vi "Begin Map by Reference.vi"(8 "Error In":errorcluster, 11 "Reader In":refnum<data-value>) -> (0 "Error Out":errorcluster, 2 "Count":u32, 3 "Reader Out":refnum<data-value>)   [LabVIEW 2017, in "LabPack.lvlib" / "Reader.lvclass"]
uses:
  Reader.lvclass
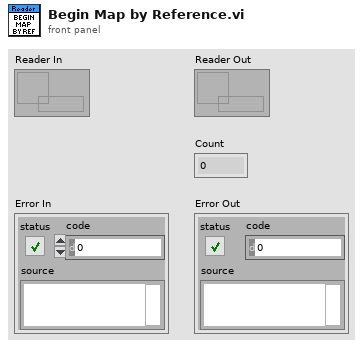
[diagram p1: front panel]
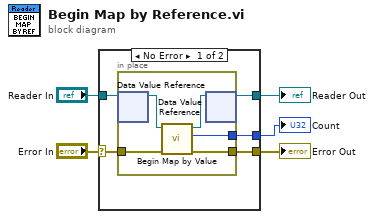
[diagram p0: block diagram]
diagram:
  n1 = case shown="No Error" "Error In" {
    selector: "Error In" -> [w8 w16]
    tunnel: "Reader In" -> [w10 w17]
    tunnel: [w9 w17] -> w4
    tunnel: [w7 w16] -> w2
    tunnel: [w6 _] -> w1
    frame No Error {
      n2 = in-place {
        in-place-border: w8 -> [w13]
        in-place-border: [w12] -> w7
        in-place-border: [w11] -> w6
        n3 = in-place-dvr #1(w10) -> (w15:refnum<class "Reader.lvclass">)  [unwired: 1 out]
        n4 = call "Begin Map by Value.vi"("Error In"=w13, "Reader In"=w15) -> ("Error Out"=w12:errorcluster, "Count"=w11:u32, "Reader Out"=w14:refnum<class "Reader.lvclass">)  [unwired: 7 in]
        n5 = in-place-dvr #1(w14) -> (w9:refnum<data-value>)  [unwired: 1 out]
      }
    }
    frame Error {
    }
  }
  "Reader Out" <- w4
  "Error Out" <- w2
  "Count" <- w1
